vi "Configure Scale Settings.vi"(0 "VISA resource name":refnum<visa-resource-name>, 1 "Y-Scale Segments (0:10 Partitions)":i32(ring) items=["10 Partitions", "12 Partitions"], 5 "Linear Scale (0:1%/div)":i32(ring) items=["1%/div", "2%/div", "5%/div", "10%/div"], 7 "Log Scale Magnification(6:10dB)":i32(ring)=6 items=["0.1 dB", "0.2 dB", "0.5 dB", "1 dB", "2 dB", "5 dB", "10 dB", "20 dB"], 9 "Unit (0:dBm)":i32(ring) items=["dBm", "dBuV", "dBmV", "dBuV (emf)", "dBuV/m", "V", "W"], 11 "error in (no error)":errorcluster, 12 "Scale Mode (0:Log Scale)":i32(ring) items=["Log Scale", "Linear Scale"]) -> (4 "VISA resource name out":refnum<visa-resource-name>, 15 "error out":errorcluster)   [LabVIEW 2020, in "Anritsu Signal Analyzer Series.lvlib"]
doc: "Configures the scale settings of the spectrum analyzer."
uses:
  Anritsu Signal Analyzer Series.lvlib
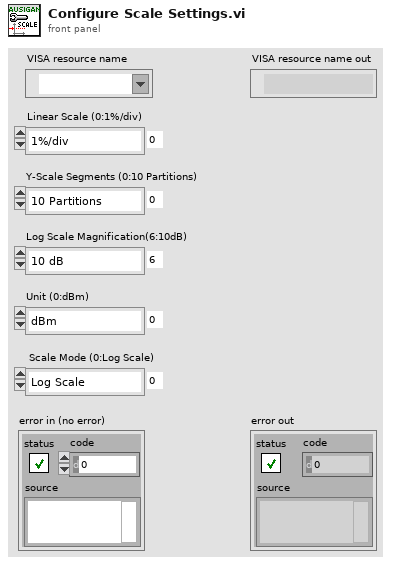
[diagram p1: front panel]
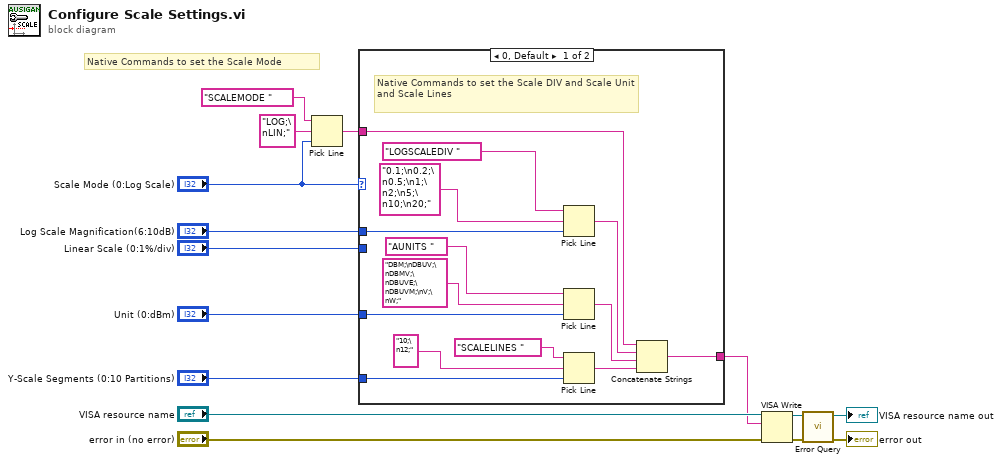
[diagram p0: block diagram]
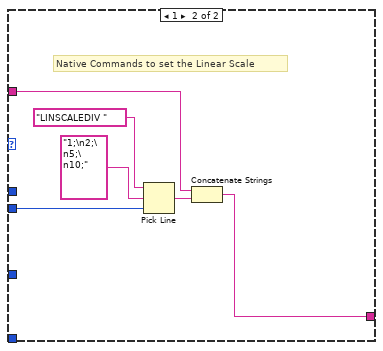
[diagram p2: hidden frame]
diagram:
  # "Native Commands to set the Scale Mode"
  n1 = Pick Line(string ("")="SCALEMODE " ("_CommandSet"), multi-line string="LOG;\nLIN;" ("複数行文字列"), line index="Scale Mode (0:Log Scale)") -> (output string=w2:string)
  n2 = case shown="0, Default" "Scale Mode (0:Log Scale)" {
    tunnel: "Log Scale Magnification(6:10dB)" -> [w27 _]
    tunnel: "Unit (0:dBm)" -> [w24 _]
    tunnel: w2 -> [w21 w31]
    tunnel: [w20 w30] -> w1
    tunnel: "Y-Scale Segments (0:10 Partitions)" -> [w17 _]
    tunnel: "Linear Scale (0:1%/div)" -> [_ w34]
    frame 0, Default {
      # "Native Commands to set the Scale DIV and Scale Unit and Scale Lines"
      n3 = Pick Line(string ("")="LOGSCALEDIV " ("_CommandSet"), multi-line string="0.1;\n0.2;\n0.5;\n1;\n2;\n5;\n10;\n20;" ("複数行文字列"), line index=w27) -> (output string=w22:string)
      n4 = Pick Line(string ("")="AUNITS " ("_CommandSet"), multi-line string="DBM;\nDBUV;\nDBMV;\nDBUVE;\nDBUVM;\nV;\nW;" ("複数行文字列"), line index=w24) -> (output string=w23:string)
      n5 = Pick Line(string ("")="SCALELINES " ("_CommandSet"), multi-line string="10;\n12;" ("複数行文字列"), line index=w17) -> (output string=w16:string)
      n6 = Concatenate Strings(w21, w22, w23, w16) -> (w20:string)
    }
    frame 1 {
      # "Native Commands to set the Linear Scale"
      n7 = Pick Line(string ("")="LINSCALEDIV " ("_CommandSet"), multi-line string="1;\n2;\n5;\n10;" ("複数行文字列"), line index=w34) -> (output string=w32:string)
      n8 = Concatenate Strings(w31, w32) -> (w30:string)
    }
  }
  n9 = VISA Write(VISA resource name="VISA resource name", write buffer=w1, error in (no error)="error in (no error)") -> (VISA resource name out=w6:refnum<visa-resource-name>, error out=w5:errorcluster)  [unwired: 1 out]
  n10 = call "Error Query.vi"("error in (no error)"=w5, "VISA resource name"=w6) -> ("error out"=→"error out":errorcluster, "VISA resource name out"=→"VISA resource name out":refnum<visa-resource-name>)  [unwired: 6 in, 2 out]
